vi "Cost.vi"(8 "error in (no error)":errorcluster, 11 "Whip in":refnum<class "Whip.lvclass">) -> (0 "error out":errorcluster, 2 "Cost":dbl, 3 "Whip out":refnum<class "Whip.lvclass">)   [LabVIEW 2013, in "Whip.lvclass"]
uses:
  Whip.lvclass
  Condiment Decorator/Condiment Decorator.lvclass
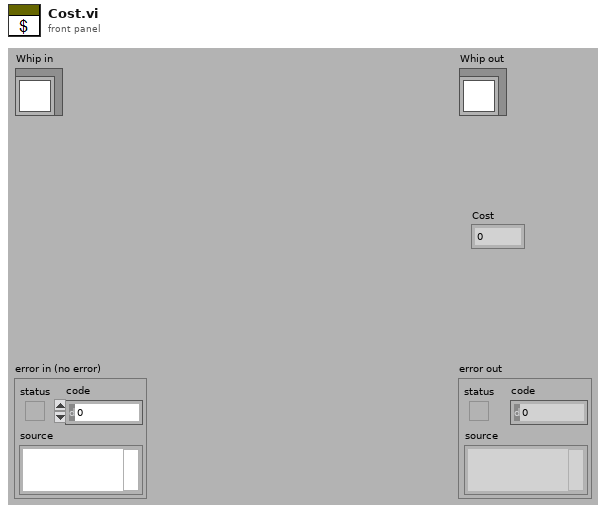
[diagram p1: front panel]
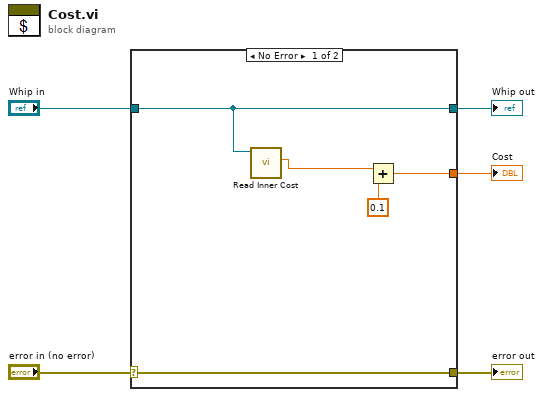
[diagram p0: block diagram]
diagram:
  n1 = case shown="No Error" "error in (no error)" {
    selector: "error in (no error)" -> [w8 w12]
    tunnel: [w8 w12] -> w4
    tunnel: [w7 w11] -> w2
    tunnel: "Whip in" -> [w7 w11]
    tunnel: [w9 _] -> w1
    frame No Error {
      n2 = call "Read Inner Cost.vi"("Condiment Decorator in"=w7) -> ("Cost"=w6:dbl)  [unwired: 10 in]
      n3 = Add(x=w6, y=0.1) -> (x+y=w9:dbl)
    }
    frame Error {
    }
  }
  "error out" <- w4
  "Whip out" <- w2
  "Cost" <- w1
